vi "VTI-RunRampT.vi"(1 "Rate (K/min)":dbl format="%#_13g", 2 "Final T (K)":dbl format="%#_13g") -> (0 "Current Setpoint":dbl format="%#_13g")   [LabVIEW 2016]
uses:
  Global/Global Variables/Data_Display_global.vi
  Instrument_Setup.vi
panel:
  out "K/s":dbl format="%#_13g"
  out "Sweep Time":dbl format="%#_13g"
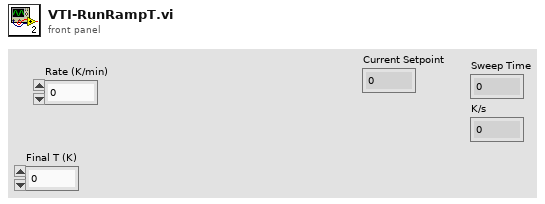
[diagram p1: front panel]
types:
  T1 = typedef "ITCIO.ctl" = cluster{"Address":T2, "Version":T3, "Ch 1 dec places":i16, "Ch 2 dec places":i16, "Ch 3 dec places":i16, "Ch1 Name":string, "Ch2 Name":string, "Ch3 Name":string}
  T2 = typedef "OxfordAddress.ctl" = cluster{"Com Port":i32, "ISOBUS Address":i32, "GPIB Address":i16, "Communication":enum16{"RS232", "ISOBUS", "GPIB", "Gateway"}}
  T3 = typedef "ITCVersion.ctl" = enum16{"ITC502", "ITC503", "ITC601"}
  T4 = typedef "VTI-cluster.ctl" = cluster{"Temperatur (K)":dbl, "Setpoint (K)":dbl, "Rate (K/min)":dbl, "Heater (%)":dbl, "NV (%)":dbl, "Heater Manual":bool, "NV Manual":bool, "Go to Set":bool, "Pressure":dbl, "Heater SP":dbl, "Valid?":bool, "Set Heater SP":bool, "Set NV SP":bool, "Heater (%) Display":dbl, "NV (%) Display":dbl, "NV Setpoint":dbl, "Change Heater Status":bool, "Change NV Status":bool, "Sample 3":dbl, "Sample 2":dbl, "Sweep-State":bool, "Set Auto PID":bool, "Auto PID":bool, "Stopp":bool, "Setpoint-Sweep":dbl}
  T5 = cluster{"ControlTITC":i8, "ControlTCh":i8, "SampleTITC":i8, "SampleTCh":i8}
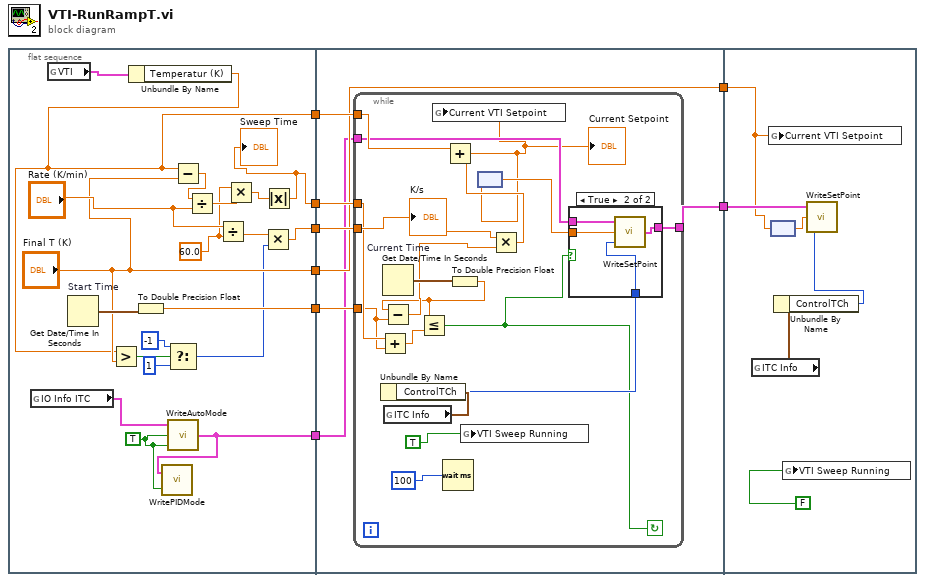
[diagram p0: block diagram]
diagram:
  n1 = flat-sequence {
    tunnel: [w10] -> w8
    tunnel: [w15] -> w7
    tunnel: [w25] -> w6
    tunnel: [w20] -> w5
    tunnel: ["Final T (K)"] -> w3
    tunnel: [w17] -> w2
    tunnel: w8 -> [w35]
    tunnel: w7 -> [w34]
    tunnel: w6 -> [w33]
    tunnel: w5 -> [w32]
    tunnel: [w31] -> w4
    tunnel: w3 -> [w31]
    tunnel: w2 -> [w30]
    tunnel: [w29] -> w1
    tunnel: w4 -> [w60]
    tunnel: w1 -> [w61]
    frame #0 {
      w18 = TRUE
      w22 = 60.0
      n2 = global read "Instrument_Setup.vi" "IO Info ITC"() -> (w19:T1)
      n3 = global read "Data_Display_global.vi" "VTI"() -> (w28:T4)
      n4 = Get Date/Time In Seconds "Start Time"() -> (seconds since 1Jan1904=w26:timestamp)
      n5 = Unbundle By Name(w28) -> ("Temperatur (K)"=w15:dbl)
      n6 = Greater?(x=w15, y="Final T (K)") -> (0:w14:bool)
      n7 = To Double Precision Float(number=w26) -> (double precision float=w25:dbl)
      n8 = Select(t=-1, s=w14, f=1) -> (s? t:f=w9:i32)
      n9 = call "WriteAutoMode.vi"("Auto Needle Valve"=w18, "Auto Heat"=w18, "ITC IO Info"=w19) -> ("ITC IO Info"=w17:T1)
      n10 = call "WritePIDMode.vi"("Auto PID"=w18, "ITC IO Info"=w17) -> ()  [unwired: 1 in, 1 out]
      n11 = Subtract(x=w15, y="Final T (K)") -> (x-y=w27:dbl)
      n12 = Divide(x=w27, y="Rate (K/min)") -> (x/y=w23:dbl)
      n13 = Divide(x="Rate (K/min)", y=w22) -> (x/y=w11:dbl)
      n14 = Multiply(x=w22, y=w23) -> (x*y=w21:dbl)
      n15 = Multiply(x=w11, y=w9) -> (x*y=w10:dbl)
      n16 = Absolute Value(x=w21) -> (abs(x)=w20:dbl)
      "Sweep Time" <- w20
    }
    frame #1 {
      n17 = while {
        tunnel: w35 -> [w51]
        tunnel: w34 -> [w48]
        tunnel: w33 -> [w39]
        tunnel: w32 -> [w47]
        tunnel: w30 -> [w42]
        tunnel: [w41] -> w29
        stop <- w38 continue-if-true
        n18 = Add(x=w47, y=w39) -> (x+y=w46:dbl)
        n19 = Get Date/Time In Seconds "Current Time"() -> (seconds since 1Jan1904=w53:timestamp)
        n20 = global read "Instrument_Setup.vi" "ITC Info"() -> (w44:T5)
        n21 = Unbundle By Name(w44) -> ("ControlTCh"=w43:i8)
        n22 = Wait (ms)(milliseconds to wait=100) -> ()  [unwired: 1 out]
        n23 = To Double Precision Float(number=w53) -> (double precision float=w40:dbl)
        n24 = Subtract(x=w40, y=w39) -> (x-y=w52:dbl)
        n25 = Less Or Equal?(x=w40, y=w46) -> (x <= y?=w38:bool)
        n26 = global write "Data_Display_global.vi" "VTI Sweep Running"(TRUE) -> ()
        n27 = Multiply(x=w51, y=w52) -> (x*y=w50:dbl)
        n28 = Add(x=w48, y=w50) -> (x+y=w37:dbl)
        "Current Setpoint" <- w37
        n29 = global write "Data_Display_global.vi" "Current VTI Setpoint"(w37) -> ()
        n30 = node(w37) -> (w45:dbl[unit])
        n31 = case shown="True" w38 {
          tunnel: w45 -> [_ w58]
          tunnel: w43 -> [_ w57]
          tunnel: w42 -> [w54 w56]
          tunnel: [w54 w55] -> w41
          frame False {
          }
          frame True {
            n32 = call "WriteSetPoint.vi"("Control Ch"=w57, "Set point"=w58, "IO Info"=w56) -> ("ITC IO Info"=w55:T1)
          }
        }
        "K/s" <- w51
      }
    }
    frame #2 {
      n33 = global read "Instrument_Setup.vi" "ITC Info"() -> (w63:T5)
      n34 = global write "Data_Display_global.vi" "Current VTI Setpoint"(w60) -> ()
      n35 = node(w60) -> (w64:dbl[unit])
      n36 = Unbundle By Name(w63) -> ("ControlTCh"=w62:i8)
      n37 = global write "Data_Display_global.vi" "VTI Sweep Running"(FALSE) -> ()
      n38 = call "WriteSetPoint.vi"("Control Ch"=w62, "Set point"=w64, "IO Info"=w61) -> ()  [unwired: 1 out]
    }
  }
